vi "TCRef.vi"(2 "offset":dbl, 3 "data":dbl) -> (0 "emf(mV)":dbl, 1 "temp (degC)":dbl)   [LabVIEW 2014]
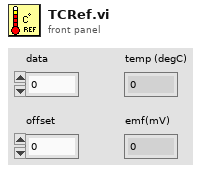
[diagram p1: front panel]
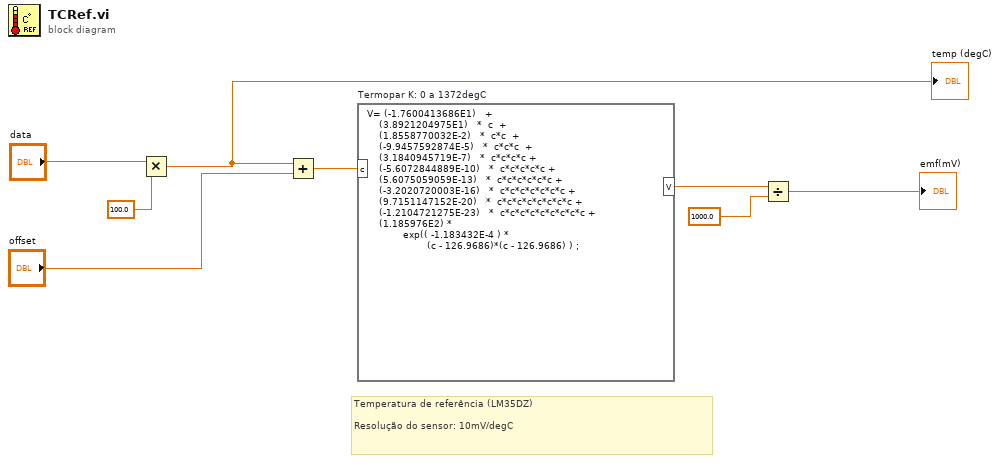
[diagram p0: block diagram]
diagram:
  # "Temperatura de referência (LM35DZ)\n\nResolução do sensor: 10mV/degC"
  n1 = Multiply(x="data", y=100.0) -> (x*y=w5:dbl)
  "temp (degC)" <- w5
  n2 = Add(x=w5, y="offset") -> (x+y=w6:dbl)
  n3 = formula code="V= (-1.7600413686E1)   +\n    (3.8921204975E1)   *  c  +\n    (1.8558770032E-2)   *  c*c  +\n    (-9.9457592874E-5)   *  c*c*c  +\n    (3.1840945719E-7)   *  c*c*c*c +\n    (-5.6072844889E-10)   *  c*c*c*c*c +\n    (5.6075059059E-13)   *  c*c*c*c*c*c +\n    (-3.2020720003E-16)   *  c*c*c*c*c*c*c +\n    (9.7151147152E-20)   *  c*c*c*c*c*c*c*c +\n    (-1.2104721275E-23)   *  c*c*c*c*c*c*c*c*c +\n    (1.185976E2) * \n            exp(( -1.183432E-4 ) * \n                    (c - 126.9686)*(c - 126.9686) ) ;" "Termopar K: 0 a 1372degC"("c"=w6) -> ("V"=w3:dbl)
  n4 = Divide(x=w3, y=1000.0) -> (x/y=→"emf(mV)":dbl)
